vi "日期范围生成-系统版.vi"(6 "单位":enum16{"年", "月", "日", "时", "分"}(ring)=enum."日" caption="单位（日）", 7 "方向":enum16{"当前", "日期+", "日期-"}(ring) caption="方向（当前）", 10 "变化量(1)":u16=1, 11 "日期时间记录":T1) -> (0 "下限":T1 caption="时间下限(时间点)", 3 "上限":T1 caption="时间上限")   [LabVIEW 2017]
uses:
  <vilib>/Utility/miscctls.llb/LVDateTimeRec.ctl
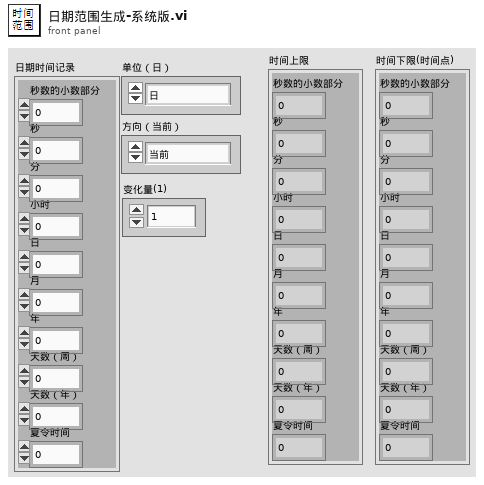
[diagram p1: front panel]
types:
  T1 = typedef "LVDateTimeRec.ctl" = cluster{"fractional second":dbl, "second":i32, "minute":i32, "hour":i32, "day of month":i32, "month":i32, "year":i32, "day of week":i32, "day of year":i32, "DST":i32}
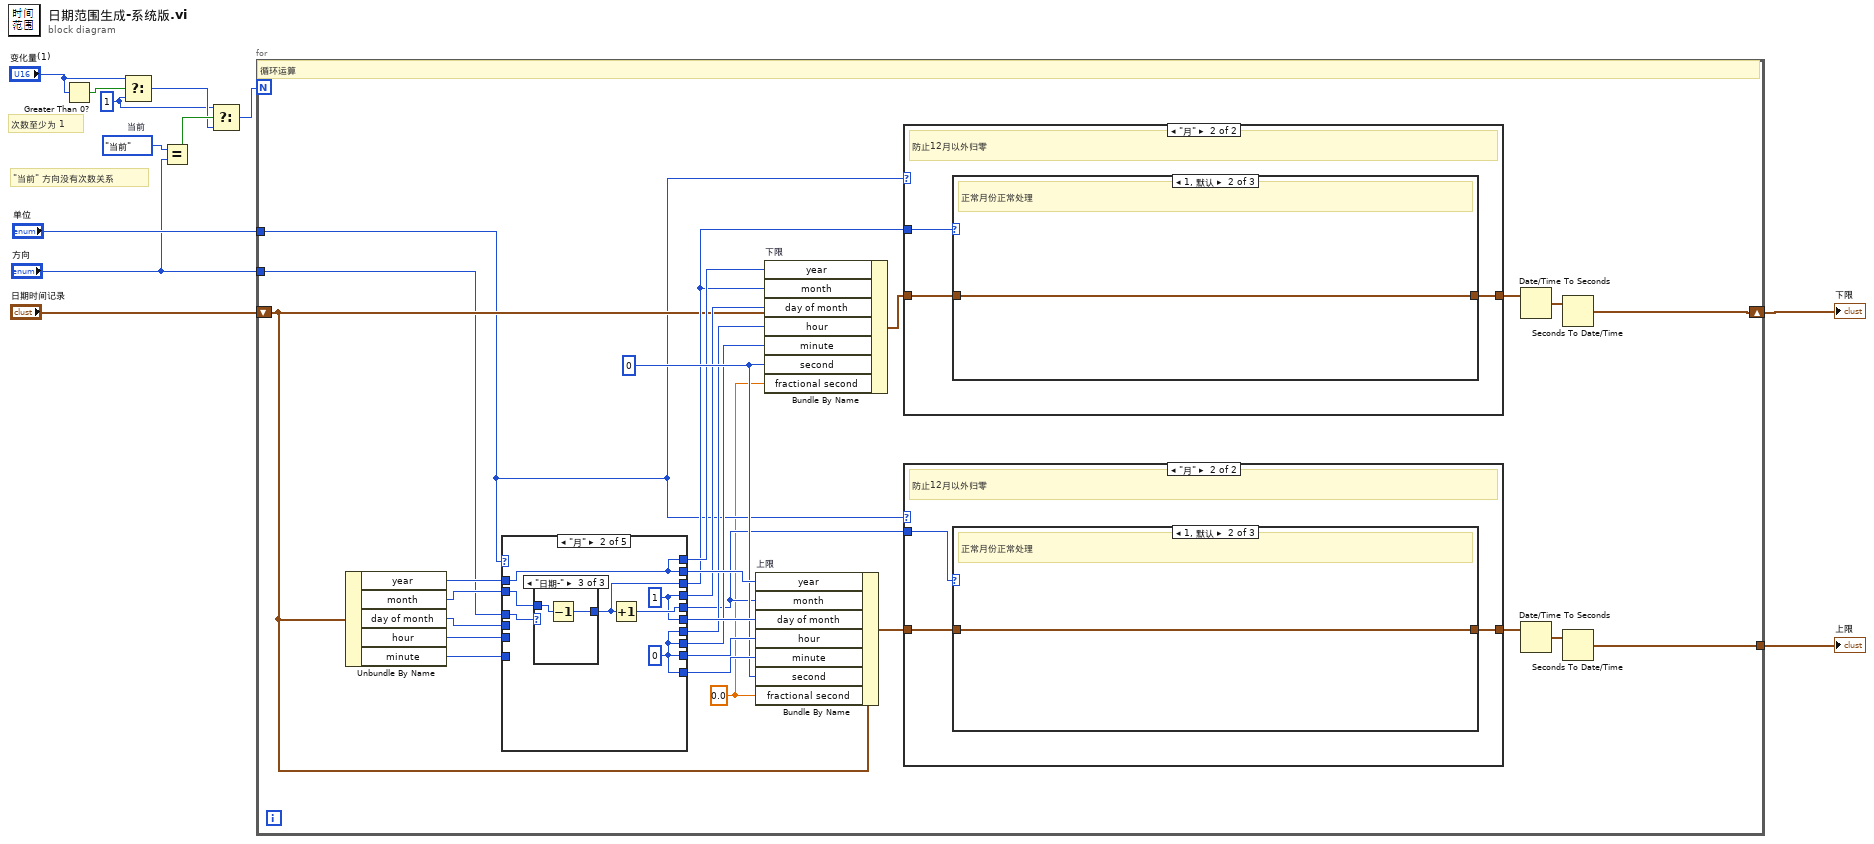
[diagram p0: block diagram]
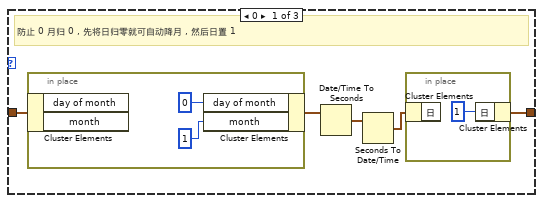
[diagram p3: hidden frame]
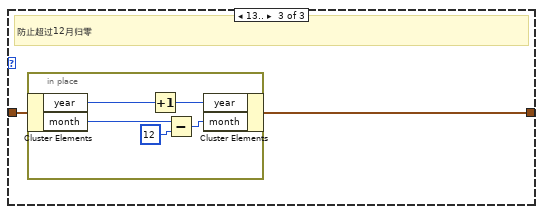
[diagram p4: hidden frame]
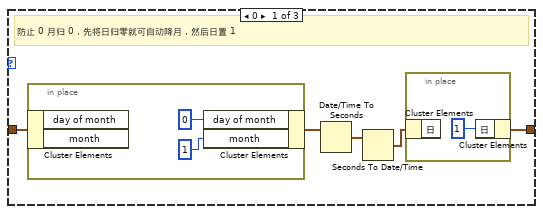
[diagram p6: hidden frame]
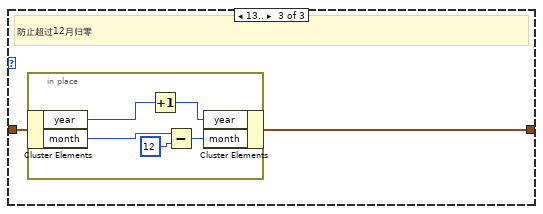
[diagram p7: hidden frame]
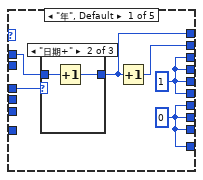
[diagram p8: hidden frame]
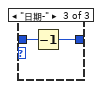
[diagram p10: hidden frame]
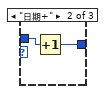
[diagram p12: hidden frame]
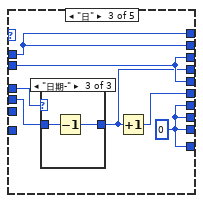
[diagram p13: hidden frame]
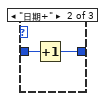
[diagram p15: hidden frame]
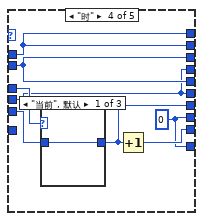
[diagram p16: hidden frame]
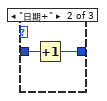
[diagram p17: hidden frame]
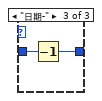
[diagram p18: hidden frame]
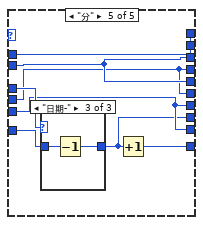
[diagram p19: hidden frame]
diagram:
  w6 = enum16{"当前", "日期+", "日期-"}."当前"  # 当前
  w3 = u16 1 ("f")
  # "\"当前\" 方向没有次数关系"
  # "次数至少为 1"
  n1 = Greater Than 0?(x="变化量(1)") -> (x > 0?=w10:bool)
  n2 = Select(t="变化量(1)", s=w10, f=w3) -> (s? t:f=w4:u16)
  n3 = Equal?(x=w6, y="方向") -> (x = y?=w5:bool)
  n4 = Select(t=w3, s=w5, f=w4) -> (s? t:f=w2:u16)
  n5 = for {
    N: w2 -> [_]
    tunnel: [w17] -> w11
    shift-right: [w14] -> w1
    shift-left: "日期时间记录" -> [w18]
    tunnel: "单位" -> [w16]
    tunnel: "方向" -> [w15]
    w13 = 0.0 ("fractional second")
    w31 = u16 0
    # "循环运算"
    n6 = Unbundle By Name(w18) -> ("year"=w39:i32, "month"=w38:i32, "day of month"=w36:i32, "hour"=w34:i32, "minute"=w32:i32)
    n7 = case shown="\"月\"" w16 {
      tunnel: [w83 w94 w107 w120 w133] -> w40
      tunnel: w39 -> [w86 w94 w107 w120 w133]
      tunnel: [w82 w96 w106 w119 w132] -> w20
      tunnel: w38 -> [_ w98 w106 w119 w132]
      tunnel: [w82 w95 w108 w118 w131] -> w37
      tunnel: w36 -> [_ _ w110 w118 w131]
      tunnel: [w81 w92 w104 w121 w130] -> w35
      tunnel: w34 -> [_ _ _ w123 w130]
      tunnel: [w81 w92 w104 w116 w134] -> w33
      tunnel: w32 -> [_ _ _ _ w135]
      tunnel: w15 -> [w85 w97 w109 w122 w136]
      tunnel: [w84 w94 w107 w120 w133] -> w30
      tunnel: [w82 w93 w106 w119 w132] -> w22
      tunnel: [w82 w95 w105 w118 w131] -> w29
      tunnel: [w81 w92 w104 w117 w130] -> w28
      tunnel: [w81 w92 w104 w116 w129] -> w27
      frame "年", Default {
        w81 = u16 0
        w82 = u16 1
        n8 = case shown="\"日期+\"" w85 {
          tunnel: [w87 w88 w90] -> w84
          tunnel: w86 -> [w87 w89 w91]
          frame "当前", Default {
          }
          frame "日期+" {
            n9 = Increment(x=w89) -> (x+1=w88:i32)
          }
          frame "日期-" {
            n10 = Decrement(x=w91) -> (x-1=w90:i32)
          }
        }
        n11 = Increment(x=w84) -> (x+1=w83:i32)
      }
      frame "月" {
        w92 = u16 0
        w95 = u16 1
        n12 = case shown="\"日期-\"" w97 {
          tunnel: [w99 w100 w102] -> w93
          tunnel: w98 -> [w99 w101 w103]
          frame "当前", Default {
          }
          frame "日期+" {
            n13 = Increment(x=w101) -> (x+1=w100:i32)
          }
          frame "日期-" {
            n14 = Decrement(x=w103) -> (x-1=w102:i32)
          }
        }
        n15 = Increment(x=w93) -> (x+1=w96:i32)
      }
      frame "日" {
        w104 = u16 0
        n16 = case shown="\"日期-\"" w109 {
          tunnel: [w111 w112 w114] -> w105
          tunnel: w110 -> [w111 w113 w115]
          frame "当前", Default {
          }
          frame "日期+" {
            n17 = Increment(x=w113) -> (x+1=w112:i32)
          }
          frame "日期-" {
            n18 = Decrement(x=w115) -> (x-1=w114:i32)
          }
        }
        n19 = Increment(x=w105) -> (x+1=w108:i32)
      }
      frame "时" {
        w116 = u16 0
        n20 = case shown="\"当前\", 默认" w122 {
          tunnel: [w124 w125 w127] -> w117
          tunnel: w123 -> [w124 w126 w128]
          frame "当前", Default {
          }
          frame "日期+" {
            n21 = Increment(x=w126) -> (x+1=w125:i32)
          }
          frame "日期-" {
            n22 = Decrement(x=w128) -> (x-1=w127:i32)
          }
        }
        n23 = Increment(x=w117) -> (x+1=w121:i32)
      }
      frame "分" {
        n24 = case shown="\"日期-\"" w136 {
          tunnel: [w137 w138 w140] -> w129
          tunnel: w135 -> [w137 w139 w141]
          frame "当前", Default {
          }
          frame "日期+" {
            n25 = Increment(x=w139) -> (x+1=w138:i32)
          }
          frame "日期-" {
            n26 = Decrement(x=w141) -> (x-1=w140:i32)
          }
        }
        n27 = Increment(x=w129) -> (x+1=w134:i32)
      }
    }
    n28 = Bundle By Name "上限"(cluster=w18, "year"=w40, "month"=w20, "day of month"=w37, "hour"=w35, "minute"=w33, "second"=w31, "fractional second"=w13) -> (w21:T1)
    n29 = Bundle By Name "下限"(cluster=w18, "year"=w30, "month"=w22, "day of month"=w29, "hour"=w28, "minute"=w27, "second"=w31, "fractional second"=w13) -> (w24:T1)
    n30 = case shown="\"月\"" w16 {
      tunnel: w24 -> [w61 w64]
      tunnel: [w61 w63] -> w23
      tunnel: w22 -> [_ w62]
      frame "年", Default {
      }
      frame "月" {
        # "防止12月以外归零"
        n31 = case shown="1, 默认" w62 {
          tunnel: w64 -> [w69 w73 w75]
          tunnel: [w66 w73 w74] -> w63
          frame 0 {
            # "防止 0 月归 0 , 先将日归零就可自动降月 , 然后日置 1"
            n32 = in-place {
              n33 = in-place-cluster #1(w69) -> ()  [unwired: 2 out]
              n34 = in-place-cluster #1("day of month"=0 ("month"), "month"=1) -> (w67:T1)
            }
            n35 = Date/Time To Seconds(2:w67) -> (0:w68:timestamp)  [unwired: 1 in]
            n36 = Seconds To Date/Time(time stamp (now)=w68) -> (date time rec=w65:T1)  [unwired: 1 in]
            n37 = in-place {
              n38 = in-place-cluster #2(w65) -> ()  [unwired: 1 out]
              n39 = in-place-cluster #2("日"=1 ("month")) -> (w66:T1)
            }
          }
          frame 1, Default {
            # "正常月份正常处理"
          }
          frame 13.. {
            # "防止超过12月归零"
            n40 = in-place {
              n41 = in-place-cluster #3(w75) -> ("year"=w80:i32, "month"=w78:i32)
              n42 = Increment(x=w80) -> (x+1=w79:i32)
              n43 = Subtract(x=w78, y=12 ("month")) -> (x-y=w76:i32)
              n44 = in-place-cluster #3("year"=w79, "month"=w76) -> (w74:T1)
            }
          }
        }
      }
    }
    n45 = case shown="\"月\"" w16 {
      tunnel: w21 -> [w41 w44]
      tunnel: [w41 w43] -> w19
      tunnel: w20 -> [_ w42]
      frame "年", Default {
      }
      frame "月" {
        # "防止12月以外归零"
        n46 = case shown="1, 默认" w42 {
          tunnel: w44 -> [w49 w53 w55]
          tunnel: [w46 w53 w54] -> w43
          frame 0 {
            # "防止 0 月归 0 , 先将日归零就可自动降月 , 然后日置 1"
            n47 = in-place {
              n48 = in-place-cluster #4(w49) -> ()  [unwired: 2 out]
              n49 = in-place-cluster #4("day of month"=0 ("month"), "month"=1) -> (w47:T1)
            }
            n50 = Date/Time To Seconds(2:w47) -> (0:w48:timestamp)  [unwired: 1 in]
            n51 = Seconds To Date/Time(time stamp (now)=w48) -> (date time rec=w45:T1)  [unwired: 1 in]
            n52 = in-place {
              n53 = in-place-cluster #5(w45) -> ()  [unwired: 1 out]
              n54 = in-place-cluster #5("日"=1 ("month")) -> (w46:T1)
            }
          }
          frame 1, Default {
            # "正常月份正常处理"
          }
          frame 13.. {
            # "防止超过12月归零"
            n55 = in-place {
              n56 = in-place-cluster #6(w55) -> ("year"=w60:i32, "month"=w57:i32)
              n57 = Increment(x=w60) -> (x+1=w59:i32)
              n58 = Subtract(x=w57, y=12 ("month")) -> (x-y=w56:i32)
              n59 = in-place-cluster #6("year"=w59, "month"=w56) -> (w54:T1)
            }
          }
        }
      }
    }
    n60 = Date/Time To Seconds(2:w23) -> (0:w26:timestamp)  [unwired: 1 in]
    n61 = Date/Time To Seconds(2:w19) -> (0:w25:timestamp)  [unwired: 1 in]
    n62 = Seconds To Date/Time(time stamp (now)=w26) -> (date time rec=w14:T1)  [unwired: 1 in]
    n63 = Seconds To Date/Time(time stamp (now)=w25) -> (date time rec=w17:T1)  [unwired: 1 in]
  }
  "上限" <- w11
  "下限" <- w1
